vi "MedianFilter2D.vi"(9 "Operation":u16(ring) items=["Median", "Mean"], 10 "Pts to use":dbl=3.0, 11 "Raw In":sgl[][](array[numeric])) -> (3 "output array":sgl[][](array[numeric]))   [LabVIEW 2022 SP3]
uses:
  <vilib>/Analysis/baseanly.llb/Mean (DBL).vi
  <vilib>/Analysis/NI_AALBase.lvlib
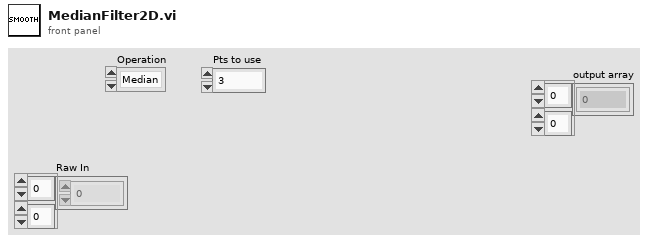
[diagram p1: front panel]
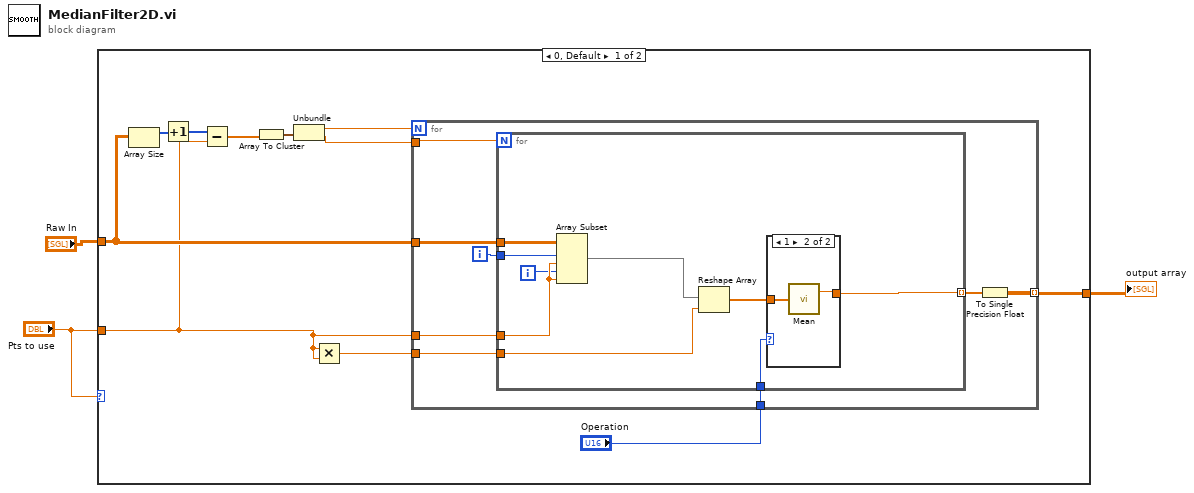
[diagram p0: block diagram]
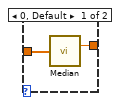
[diagram p2: hidden frame]
diagram:
  n1 = case shown="0, Default" "Pts to use" {
    tunnel: "Pts to use" -> [w6 _]
    tunnel: "Raw In" -> [w7 w36]
    tunnel: [w5 w36] -> w2
    frame 0, Default {
      n2 = Array Size(array=w7) -> (size(s)=w8:i32[])
      n3 = Increment(x=w8) -> (x+1=w4:i32[])
      n4 = Subtract(x=w4, y=w6) -> (x-y=w9:dbl[])
      n5 = Array To Cluster(array=w9) -> (cluster=w12:cluster{"[0]":dbl, "[1]":dbl})
      n6 = Unbundle(w12) -> ("[0]"=w11:dbl, "[1]"=w10:dbl)
      n7 = Multiply(x=w6, y=w6) -> (x*y=w14:dbl)
      n8 = for {
        N: w11 -> [_]
        tunnel: w7 -> [w22]
        tunnel: w6 -> [w21]
        tunnel: w14 -> [w20]
        tunnel: [w18] -> w5 mode=indexing
        tunnel: "Operation" -> [w17]
        tunnel: w10 -> [w16]
        i -> [w15]
        n9 = for {
          N: w16 -> [_]
          tunnel: w22 -> [w31]
          tunnel: w21 -> [w30]
          tunnel: w15 -> [w25]
          tunnel: w20 -> [w28]
          tunnel: [w26] -> w19 mode=indexing
          tunnel: w17 -> [w24]
          i -> [w23]
          n10 = Array Subset(array=w31, index (row)=w25, length (row)=w30, index (col)=w23, length (col)=w30) -> (w29:sgl[][])
          n11 = Reshape Array(w29, w28) -> (w27:sgl[])
          n12 = case shown="1" w24 {
            tunnel: w27 -> [w33 w35]
            tunnel: [w32 w34] -> w26
            frame 0, Default {
              n13 = call <vilib>:"Median.vi"("X"=w33) -> ("median"=w32:dbl)  [unwired: 1 out]
            }
            frame 1 {
              n14 = call-poly <vilib>:"Mean.vi"("X"=w35) -> ("mean"=w34:dbl)  [unwired: 1 out]
            }
          }
        }
        n15 = To Single Precision Float(number=w19) -> (single precision float=w18:sgl[])
      }
    }
    frame 1 {
    }
  }
  "output array" <- w2
